vi "Calc_TipperV2.vi"(8 "Desired Voltage":dbl, 9 "PID":T1={"proportional gain (Kc)"=1.0, "integral time (Ti, min)"=0.0, "derivative time (Td, min)"=0.0} {"derivative time (Td, min)" format="%.3f"; "integral time (Ti, min)" format="%.3f"; "proportional gain (Kc)" format="%.3f"}, 10 "Tipper Inputs":T2, 11 "Tipper Command Inputs":T3) -> (0 "dt out (s)":dbl format="%.3f", 3 "Bridge Tipper Outputs":T4)   [LabVIEW 2011]
uses:
  Outputs_Tipper.ctl
  Inputs_TipperV2.ctl
  Inputs_Sensors_TipperV2.ctl
  <vilib>/addons/control/pid/pid.llb/PID (DBL).vi
  <vilib>/addons/control/pid/NI_PID_pid.lvlib
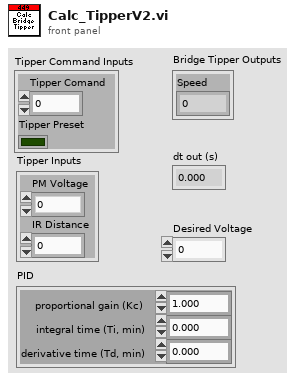
[diagram p1: front panel]
types:
  T1 = cluster{"proportional gain (Kc)":dbl, "integral time (Ti, min)":dbl, "derivative time (Td, min)":dbl}
  T2 = typedef "Inputs_Sensors_TipperV2.ctl" = cluster{"PM Voltage":dbl, "IR Distance":dbl}
  T3 = typedef "Inputs_TipperV2.ctl" = cluster{"Tipper Comand":dbl, "Tipper Preset":bool}
  T4 = typedef "Outputs_Tipper.ctl" = cluster{"Speed":dbl}
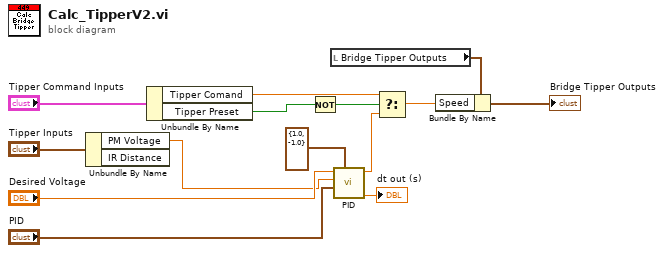
[diagram p0: block diagram]
diagram:
  n1 = Unbundle By Name("Tipper Inputs") -> ("PM Voltage"=w1:dbl)  [unwired: 1 out]
  n2 = Unbundle By Name("Tipper Command Inputs") -> ("Tipper Comand"=w4:dbl, "Tipper Preset"=w8:bool)
  n3 = Not(x=w8) -> (.not. x?=w7:bool)
  n4 = local read "Bridge Tipper Outputs"() -> (w14:T4)
  n5 = call-poly <vilib>:"PID.vi"("output range"=cluster{"output high":dbl, "output low":dbl} {"output high"=1.0, "output low"=-1.0}, "PID gains"="PID", "process variable"=w1, "setpoint"="Desired Voltage") -> ("dt out (s)"=→"dt out (s)":dbl, "output"=w6:dbl)  [unwired: 6 in]
  n6 = Select(t=w4, s=w7, f=w6) -> (s? t:f=w9:dbl)
  n7 = Bundle By Name(cluster=w14, "Speed"=w9) -> (→"Bridge Tipper Outputs":T4)
